vi "projectorXY2CameraXY.vi"(9 "Linear Transformation Description Template":T1 {"mean error\n(projector pixels)" format="%0.2f"}, 11 "Projector Point":cluster{"X":sgl, "Y":sgl} {"Y" format="%.2f"; "X" format="%.2f"}) -> (3 "Camera Point":cluster{"X":sgl, "Y":sgl} {"Y" format="%.2f"; "X" format="%.2f"})   [LabVIEW 2019]
uses:
  LinearTransformationDescriptionCluster.ctl
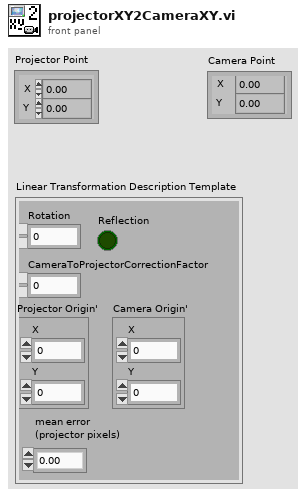
[diagram p1: front panel]
types:
  T1 = typedef "LinearTransformationDescriptionCluster.ctl" = cluster{"Rotation":sgl, "Reflection":bool, "CameraToProjectorCorrectionFactor":dbl, "Projector Origin'":cluster{"X":dbl, "Y":dbl}, "Camera Origin'":cluster{"X":dbl, "Y":dbl}, "mean error\n(projector pixels)":dbl}
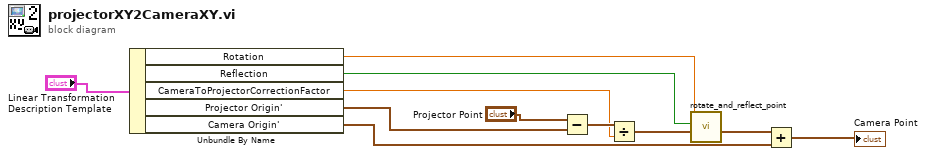
[diagram p0: block diagram]
diagram:
  n1 = Unbundle By Name("Linear Transformation Description Template") -> ("Rotation"=w6:sgl, "Reflection"=w5:bool, "CameraToProjectorCorrectionFactor"=w3:dbl, "Projector Origin'"=w4:cluster{"X":dbl, "Y":dbl}, "Camera Origin'"=w2:cluster{"X":dbl, "Y":dbl})
  n2 = Subtract(x="Projector Point", y=w4) -> (x-y=w10:cluster{"X":dbl, "Y":dbl})
  n3 = Divide(x=w10, y=w3) -> (x/y=w9:cluster{"X":dbl, "Y":dbl})
  n4 = call "rotate_and_reflect_point.vi"("Point"=w9, "reflect about the x axis?"=w5, "rotation angle (radians)"=w6) -> ("transformed point"=w8:cluster{"X":sgl, "Y":sgl})  [unwired: 8 in]
  n5 = Add(x=w8, y=w2) -> (x+y=→"Camera Point":cluster{"X":dbl, "Y":dbl})
